vi "Get Pane Bounds.vi"(8 "error in (no error)":errorcluster, 11 "Pane":refnum<vi>) -> (0 "error out":errorcluster, 3 "Panel Coordinates":T1)   [LabVIEW 2018, in "Pane Object Position.lvclass"]
uses:
  Pane Object Position.lvclass
  Object Coordinates.ctl
  <vilib>/Utility/miscctls.llb/LVPointTypeDef.ctl
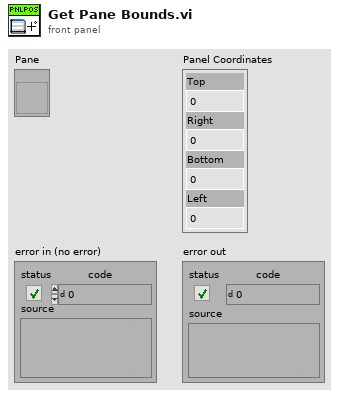
[diagram p1: front panel]
types:
  T1 = typedef "Pane Object Position.lvclass/Object Coordinates.ctl" = cluster{"Top":i32, "Right":i32, "Bottom":i32, "Left":i32}
  T2 = typedef "LVPointTypeDef.ctl" = cluster{"Horizontal":i16, "Vertical":i16}
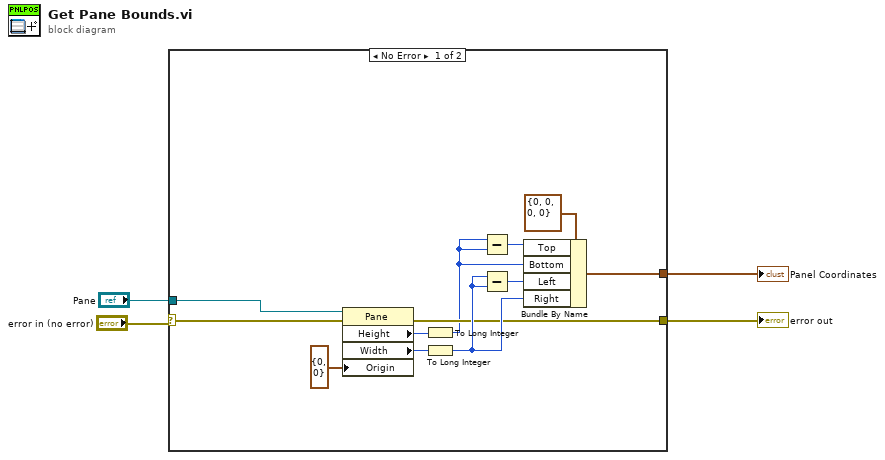
[diagram p0: block diagram]
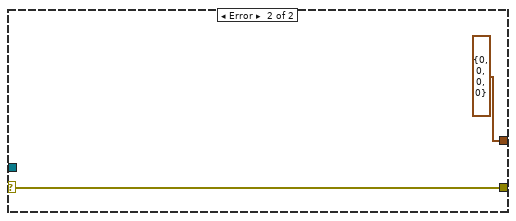
[diagram p2: hidden frame]
diagram:
  n1 = case shown="No Error" "error in (no error)" {
    selector: "error in (no error)" -> [w8 w17]
    tunnel: [w9 T1 {"Top"=0, "Right"=0, "Bottom"=0, "Left"=0} ("output cluster")] -> w4
    tunnel: [w7 w17] -> w2
    tunnel: "Pane" -> [w5 _]
    frame No Error {
      n2 = property class="Pane"(reference=w5, error in=w8, "Origin"=T2 {"Horizontal"=0, "Vertical"=0}) -> (error out=w7:errorcluster, "Height"=w16:u32, "Width"=w15:u32)  [unwired: 1 out]
      n3 = To Long Integer(number=w16) -> (32bit integer=w6:i32)
      n4 = To Long Integer(number=w15) -> (32bit integer=w12:i32)
      n5 = Subtract(x=w6, y=w6) -> (x-y=w14:i32)
      n6 = Subtract(x=w12, y=w12) -> (x-y=w13:i32)
      n7 = Bundle By Name(cluster=T1 {"Top"=0, "Right"=0, "Bottom"=0, "Left"=0} ("output cluster"), "Top"=w14, "Bottom"=w6, "Left"=w13, "Right"=w12) -> (w9:T1)
    }
    frame Error {
    }
  }
  "Panel Coordinates" <- w4
  "error out" <- w2
